vi "player.vi"() -> ()   [LabVIEW 2012]
uses:
  <vilib>/Utility/error.llb/DialogType.ctl
  player_glo.vi
  musicplayer_glo.vi
panel:
  in  "WindowsMediaPlayer":refnum<k7>(container)
  # "(c) Aron Heinecke 2013\nsupport.proctet@t-online.de"
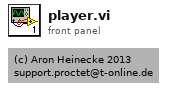
[diagram p1: front panel]
types:
  T1 = typedef "DialogType.ctl" = u16
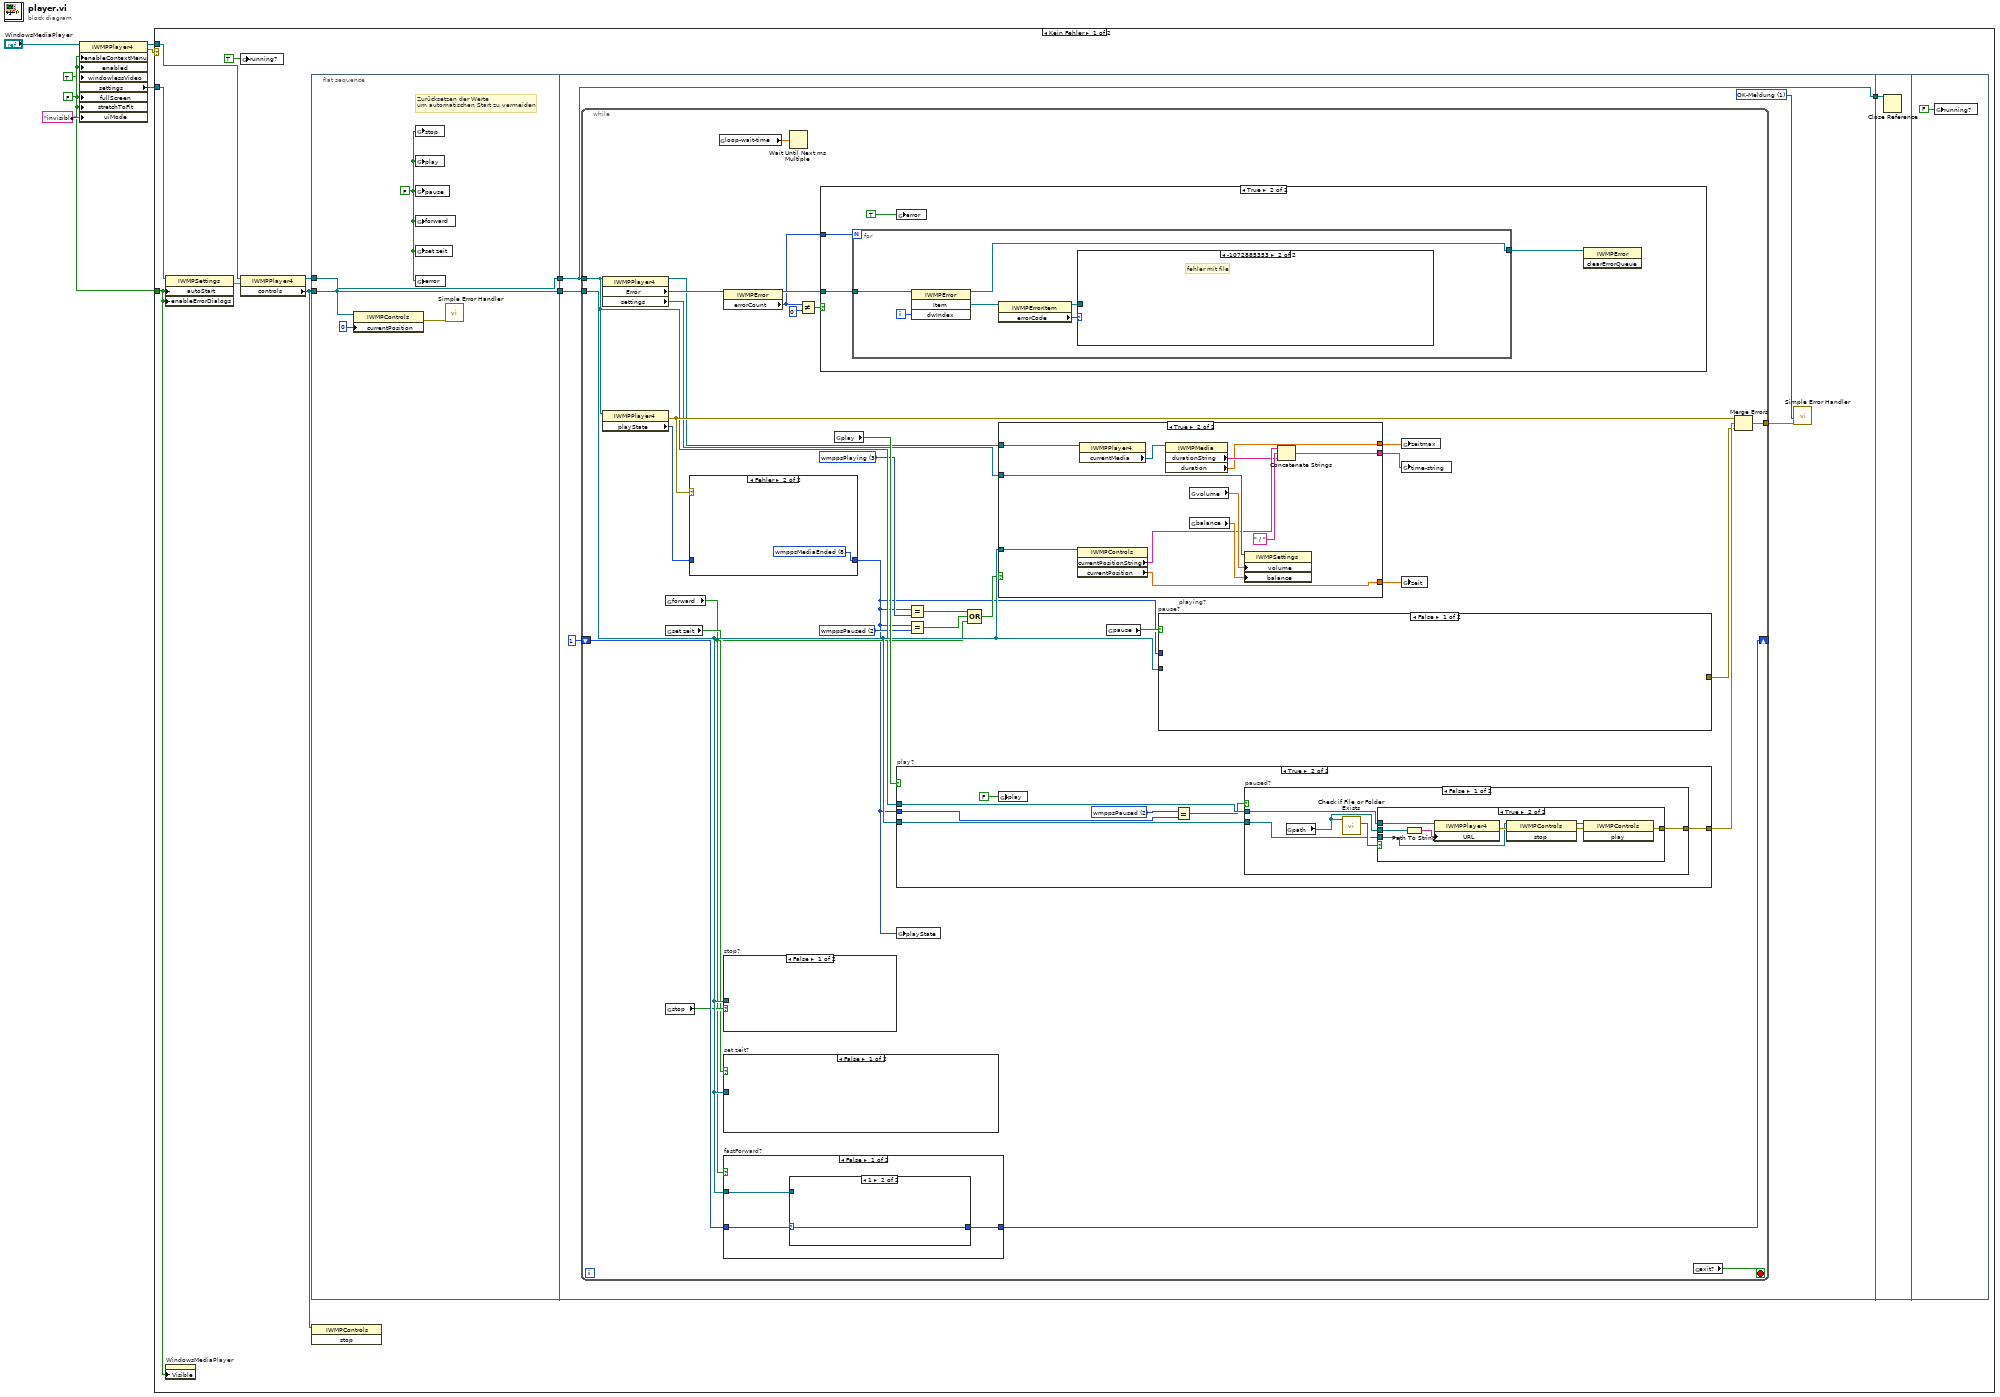
[diagram p0: block diagram]
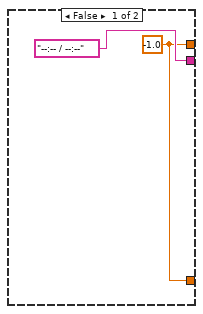
[diagram p2: hidden frame]
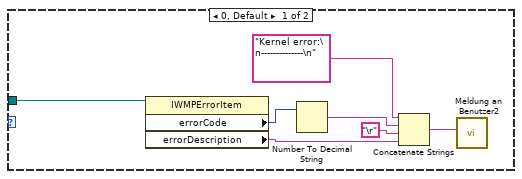
[diagram p4: hidden frame]
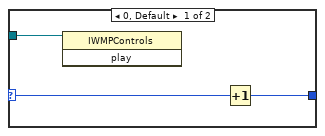
[diagram p6: hidden frame]
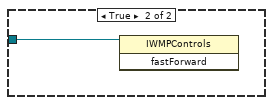
[diagram p7: hidden frame]
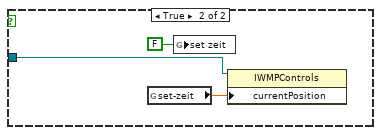
[diagram p8: hidden frame]
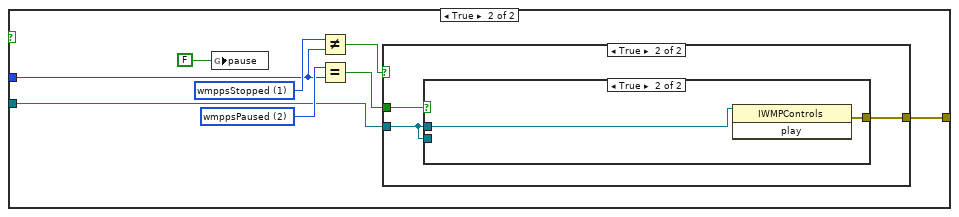
[diagram p9: hidden frame]
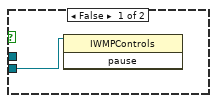
[diagram p11: hidden frame]
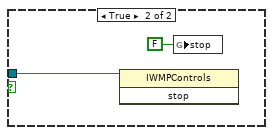
[diagram p12: hidden frame]
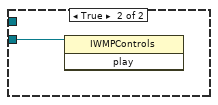
[diagram p15: hidden frame]
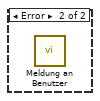
[diagram p16: hidden frame]
diagram:
  w3 = FALSE ("enableContextMenu")
  n1 = property class="IWMPPlayer4"(reference="WindowsMediaPlayer", "enableContextMenu"=w3, "enabled"=w3, "windowlessVideo"=TRUE, "fullScreen"=w3, "stretchToFit"=w3, "uiMode"="invisible") -> (reference out=w1:refnum<k7>, error out=w5:errorcluster, "settings"=w4:refnum<k7>)  [unwired: 1 in]
  n2 = case shown="Kein Fehler" w5 {
    tunnel: w4 -> [w11 _]
    tunnel: w3 -> [w9 _]
    tunnel: w1 -> [w8 _]
    frame No Error {
      n3 = property class="IWMPSettings"(reference=w11, "autoStart"=w9, "enableErrorDialogs"=w9) -> (error out=w17:errorcluster)  [unwired: 1 in, 1 out]
      n4 = property on="WindowsMediaPlayer" class="AXCont"("Visible"=w9) -> ()  [unwired: 2 in, 2 out]
      n5 = global write "player_glo.vi" "running?"(TRUE ("windowlessVideo")) -> ()
      n6 = property class="IWMPPlayer4"(reference=w8, error in=w17) -> (reference out=w16:refnum<k7>, "controls"=w14:refnum<k7>)  [unwired: 1 out]
      n7 = flat-sequence {
        tunnel: w14 -> [w20]
        tunnel: w16 -> [w22]
        tunnel: [w22] -> w13
        tunnel: [w20] -> w12
        tunnel: [w26] -> w15
        tunnel: w13 -> [w26]
        tunnel: w12 -> [w27]
        tunnel: w15 -> [w141]
        frame #0 {
          w21 = FALSE
          # "Zurücksetzen der Werte\num automatischen Start zu vermeiden"
          n8 = property class="IWMPControls"(reference=w20, "currentPosition"=0) -> (error out=w18:errorcluster)  [unwired: 1 in, 1 out]
          n9 = global write "player_glo.vi" "stop"(w21) -> ()
          n10 = global write "player_glo.vi" "play"(w21) -> ()
          n11 = global write "player_glo.vi" "pause"(w21) -> ()
          n12 = global write "player_glo.vi" "forward"(w21) -> ()
          n13 = global write "player_glo.vi" "set zeit"(w21) -> ()
          n14 = global write "player_glo.vi" "error"(w21) -> ()
          n15 = call <vilib>:"Simple Error Handler.vi"("error in (no error)"=w18) -> ()  [unwired: 4 in, 5 out]
        }
        frame #1 {
          w23 = T1 1 items=["Kein Dialog", "OK-Meldung", "Dialog zum Fortsetzen oder Anhalten", "OK-Meldung + Warnungen", "Weiter/Stopp + Warnung"] ("type of dialog (OK msg:1)")
          n16 = while {
            tunnel: w26 -> [w49]
            tunnel: w27 -> [w54]
            shift-right: [w55] -> _
            shift-left: 1 -> [w56]
            tunnel: [w50] -> w24
            stop <- w59 stop-if-true
            w44 = 2 items=["wmppsUndefined", "wmppsStopped", "wmppsPaused", "wmppsPlaying", "wmppsScanForward", "wmppsScanReverse", "wmppsBuffering", "wmppsWaiting", "wmppsMediaEnded", "wmppsTransitioning", "wmppsReady", "wmppsReconnecting", "wmppsLast"] ("playState")
            w46 = 3 items=["wmppsUndefined", "wmppsStopped", "wmppsPaused", "wmppsPlaying", "wmppsScanForward", "wmppsScanReverse", "wmppsBuffering", "wmppsWaiting", "wmppsMediaEnded", "wmppsTransitioning", "wmppsReady", "wmppsReconnecting", "wmppsLast"] ("playState")
            n17 = property class="IWMPPlayer4"(reference=w49) -> (reference out=w35:refnum<k7>, "Error"=w38:refnum<k7>, "settings"=w37:refnum<k7>)  [unwired: 1 in, 1 out]
            n18 = property class="IWMPPlayer4"(reference=w49) -> (error out=w53:errorcluster, "playState"=w39:i32)  [unwired: 1 in, 1 out]
            n19 = global read "player_glo.vi" "forward"() -> (w41:bool)
            n20 = global read "player_glo.vi" "set zeit"() -> (w42:bool)
            n21 = global read "player_glo.vi" "stop"() -> (w48:bool)
            n22 = case shown="Fehler" w53 {
              tunnel: [w91 w92] -> w40
              tunnel: w39 -> [w91 _]
              frame No Error {
              }
              frame Error {
                w92 = 8 items=["wmppsUndefined", "wmppsStopped", "wmppsPaused", "wmppsPlaying", "wmppsScanForward", "wmppsScanReverse", "wmppsBuffering", "wmppsWaiting", "wmppsMediaEnded", "wmppsTransitioning", "wmppsReady", "wmppsReconnecting", "wmppsLast"] ("playState")
              }
            }
            n23 = global read "player_glo.vi" "loop-wait-time"() -> (w57:dbl)
            n24 = property class="IWMPError"(reference=w38) -> (reference out=w33:refnum<k7>, "errorCount"=w31:i32)  [unwired: 1 in, 1 out]
            n25 = case "stop?" shown="False" w48 {
              tunnel: w54 -> [_ w118]
              frame False {
              }
              frame True {
                n26 = invoke class="IWMPControls" method="stop"(reference=w118) -> ()  [unwired: 2 in, 3 out]
                n27 = global write "player_glo.vi" "stop"(FALSE) -> ()
              }
            }
            n28 = case "set zeit?" shown="False" w42 {
              tunnel: w54 -> [_ w103]
              frame False {
              }
              frame True {
                n29 = global read "player_glo.vi" "set-zeit"() -> (w102:dbl)
                n30 = global write "player_glo.vi" "set zeit"(FALSE) -> ()
                n31 = property class="IWMPControls"(reference=w103, "currentPosition"=w102) -> ()  [unwired: 1 in, 2 out]
              }
            }
            n32 = case "fastForward?" shown="False" w41 {
              tunnel: w54 -> [w95 w100]
              tunnel: w56 -> [w94 _]
              tunnel: [w93 _] -> w55
              frame False {
                n33 = case shown="1" w94 {
                  selector: w94 -> [w98 w99]
                  tunnel: w95 -> [w96 _]
                  tunnel: [w97 w99] -> w93
                  frame 0, Default {
                    n34 = invoke class="IWMPControls" method="play"(reference=w96) -> ()  [unwired: 2 in, 3 out]
                    n35 = Increment(x=w98) -> (x+1=w97:i32)
                  }
                  frame 1 {
                  }
                }
              }
              frame True {
                n36 = invoke class="IWMPControls" method="fastForward"(reference=w100) -> ()  [unwired: 2 in, 3 out]
              }
            }
            n37 = Wait Until Next ms Multiple(millisecond multiple=w57) -> ()  [unwired: 1 out]
            n38 = Not Equal?(x=w31, y=0) -> (x != y?=w34:bool)
            n39 = case shown="True" w34 {
              tunnel: w33 -> [_ w77]
              tunnel: w31 -> [_ w76]
              frame False {
              }
              frame True {
                n40 = for {
                  N: w76 -> [_]
                  tunnel: w77 -> [w83]
                  tunnel: [w78] -> w74
                  i -> [w82]
                  n41 = invoke class="IWMPError" method="Item"(reference=w83, "dwIndex"=w82) -> (reference out=w78:refnum<k7>, "Item"=w81:refnum<k7>)  [unwired: 2 in, 2 out]
                  n42 = property class="IWMPErrorItem"(reference=w81) -> (reference out=w79:refnum<k7>, "errorCode"=w80:i32)  [unwired: 1 in, 1 out]
                  n43 = case shown="-1072885353" w80 {
                    tunnel: w79 -> [w88 _]
                    frame 0, Default {
                      n44 = property class="IWMPErrorItem"(reference=w88) -> ("errorCode"=w87:i32, "errorDescription"=w84:string)  [unwired: 1 in, 2 out]
                      n45 = Number To Decimal String(number=w87) -> (decimal integer string=w86:string)  [unwired: 1 in]
                      n46 = Concatenate Strings("Kernel error:\n--------------\n" ("String"), w86, "\r", w84) -> (w90:string)
                      n47 = call "Meldung an Benutzer2"("Message"=w90) -> ()  [unwired: 9 in, 2 out]
                    }
                    frame -1072885353 {
                      # "fehler mit file"
                    }
                  }
                }
                n48 = global write "player_glo.vi" "error"(TRUE ("error")) -> ()
                n49 = invoke class="IWMPError" method="clearErrorQueue"(reference=w74) -> ()  [unwired: 2 in, 3 out]
              }
            }
            n50 = global read "player_glo.vi" "play"() -> (w58:bool)
            n51 = case "play?" shown="True" w58 {
              tunnel: w54 -> [_ w125]
              tunnel: w49 -> [_ w126]
              tunnel: w40 -> [_ w122]
              tunnel: [_ w120] -> w52
              frame False {
              }
              frame True {
                w124 = 2 items=["wmppsUndefined", "wmppsStopped", "wmppsPaused", "wmppsPlaying", "wmppsScanForward", "wmppsScanReverse", "wmppsBuffering", "wmppsWaiting", "wmppsMediaEnded", "wmppsTransitioning", "wmppsReady", "wmppsReconnecting", "wmppsLast"] ("playState")
                n52 = global write "player_glo.vi" "play"(FALSE ("play")) -> ()
                n53 = Equal?(x=w124, y=w122) -> (x = y?=w123:bool)
                n54 = case "paused?" shown="False" w123 {
                  tunnel: w126 -> [w130 _]
                  tunnel: w125 -> [w128 w140]
                  tunnel: [w127 _] -> w120
                  frame False {
                    n55 = global read "player_glo.vi" "path"() -> (w129:path)
                    n56 = call <vilib>:"Check if File or Folder Exists.vi"("path"=w129) -> ("file or folder exists?"=w131:bool)  [unwired: 8 in, 2 out]
                    n57 = case shown="True" w131 {
                      tunnel: w130 -> [_ w137]
                      tunnel: w129 -> [_ w139]
                      tunnel: w128 -> [_ w135]
                      tunnel: [_ w132] -> w127
                      frame False {
                      }
                      frame True {
                        n58 = Path To String(path=w139) -> (string=w138:string)
                        n59 = property class="IWMPPlayer4"(reference=w137, "URL"=w138) -> (error out=w136:errorcluster)  [unwired: 1 in, 1 out]
                        n60 = invoke class="IWMPControls" method="stop"(reference=w135, error in=w136) -> (reference out=w134:refnum<k7>, error out=w133:errorcluster)  [unwired: 1 in, 1 out]
                        n61 = invoke class="IWMPControls" method="play"(reference=w134, error in=w133) -> (error out=w132:errorcluster)  [unwired: 1 in, 2 out]
                      }
                    }
                  }
                  frame True {
                    n62 = invoke class="IWMPControls" method="play"(reference=w140) -> ()  [unwired: 2 in, 3 out]
                  }
                }
              }
            }
            n63 = global write "player_glo.vi" "playState"(w40) -> ()
            n64 = Equal?(x=w40, y=w46) -> (x = y?=w36:bool)
            n65 = Equal?(x=w40, y=w44) -> (x = y?=w43:bool)
            n66 = Compound Arithmetic op=OR(w36, w43, w41) -> (w45:bool)
            n67 = case "playing?" shown="True" w45 {
              tunnel: w37 -> [_ w71]
              tunnel: w54 -> [_ w70]
              tunnel: ["--:-- / --:--" w66] -> w30
              tunnel: [w60 w65] -> w29
              tunnel: [w60 w64] -> w28
              tunnel: w35 -> [_ w62]
              frame False {
                w60 = -1.0 ("currentPosition")
              }
              frame True {
                n68 = property class="IWMPControls"(reference=w70) -> ("currentPositionString"=w69:string, "currentPosition"=w65:dbl)  [unwired: 1 in, 2 out]
                n69 = property class="IWMPPlayer4"(reference=w62) -> ("currentMedia"=w63:refnum<k7>)  [unwired: 1 in, 2 out]
                n70 = property class="IWMPMedia"(reference=w63) -> ("durationString"=w67:string, "duration"=w64:dbl)  [unwired: 1 in, 2 out]
                n71 = global read "player_glo.vi" "volume"() -> (w72:dbl)
                n72 = global read "player_glo.vi" "balance"() -> (w73:dbl)
                n73 = property class="IWMPSettings"(reference=w71, "volume"=w72, "balance"=w73) -> ()  [unwired: 1 in, 2 out]
                n74 = Concatenate Strings(w69, " / ", w67) -> (w66:string)
              }
            }
            n75 = global read "player_glo.vi" "pause"() -> (w47:bool)
            n76 = case "pause?" shown="False" w47 {
              tunnel: w54 -> [_ w109]
              tunnel: w40 -> [_ w107]
              tunnel: [_ w104] -> w51
              frame False {
              }
              frame True {
                w108 = 1 items=["wmppsUndefined", "wmppsStopped", "wmppsPaused", "wmppsPlaying", "wmppsScanForward", "wmppsScanReverse", "wmppsBuffering", "wmppsWaiting", "wmppsMediaEnded", "wmppsTransitioning", "wmppsReady", "wmppsReconnecting", "wmppsLast"] ("playState")
                w110 = 2 items=["wmppsUndefined", "wmppsStopped", "wmppsPaused", "wmppsPlaying", "wmppsScanForward", "wmppsScanReverse", "wmppsBuffering", "wmppsWaiting", "wmppsMediaEnded", "wmppsTransitioning", "wmppsReady", "wmppsReconnecting", "wmppsLast"] ("playState")
                n77 = global write "player_glo.vi" "pause"(FALSE ("pause")) -> ()
                n78 = Not Equal?(x=w108, y=w107) -> (x != y?=w105:bool)
                n79 = Equal?(x=w110, y=w107) -> (x = y?=w106:bool)
                n80 = case shown="True" w105 {
                  tunnel: w109 -> [_ w114]
                  tunnel: w106 -> [_ w113]
                  tunnel: [_ w112] -> w104
                  frame False {
                  }
                  frame True {
                    n81 = case shown="True" w113 {
                      tunnel: w114 -> [_ w117]
                      tunnel: w114 -> [w115 _]
                      tunnel: [_ w116] -> w112
                      frame False {
                        n82 = invoke class="IWMPControls" method="pause"(reference=w115) -> ()  [unwired: 2 in, 3 out]
                      }
                      frame True {
                        n83 = invoke class="IWMPControls" method="play"(reference=w117) -> (error out=w116:errorcluster)  [unwired: 2 in, 2 out]
                      }
                    }
                  }
                }
              }
            }
            n84 = global write "player_glo.vi" "zeitmax"(w28) -> ()
            n85 = global write "player_glo.vi" "time-string"(w30) -> ()
            n86 = global write "player_glo.vi" "zeit"(w29) -> ()
            n87 = global read "musicplayer_glo.vi" "exit?"() -> (w59:bool)
            n88 = Merge Errors(w53, w52, w51) -> (w50:errorcluster)
          }
          n89 = call <vilib>:"Simple Error Handler.vi"("type of dialog (OK msg:1)"=w23, "error in (no error)"=w24) -> ()  [unwired: 3 in, 5 out]
        }
        frame #2 {
          n90 = Close Reference(reference=w141) -> ()  [unwired: 1 in, 1 out]
        }
        frame #3 {
          n91 = global write "player_glo.vi" "running?"(FALSE) -> ()
        }
      }
      n92 = invoke class="IWMPControls" method="stop"(reference=w14) -> ()  [unwired: 2 in, 3 out]
    }
    frame Error {
      n93 = call "Meldung an Benutzer"() -> ()  [unwired: 3 in, 9 out]
    }
  }
